vi "Common Path to Specific Path.vi"(10 "common path":string) -> (2 "specific path":path)   [LabVIEW 2020, in "NI_LVConfig.lvlib"]
uses:
  <vilib>/Utility/config.llb/NI_LVConfig.lvlib
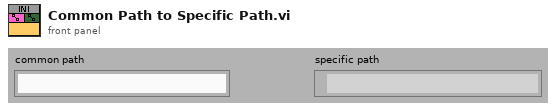
[diagram p1: front panel]
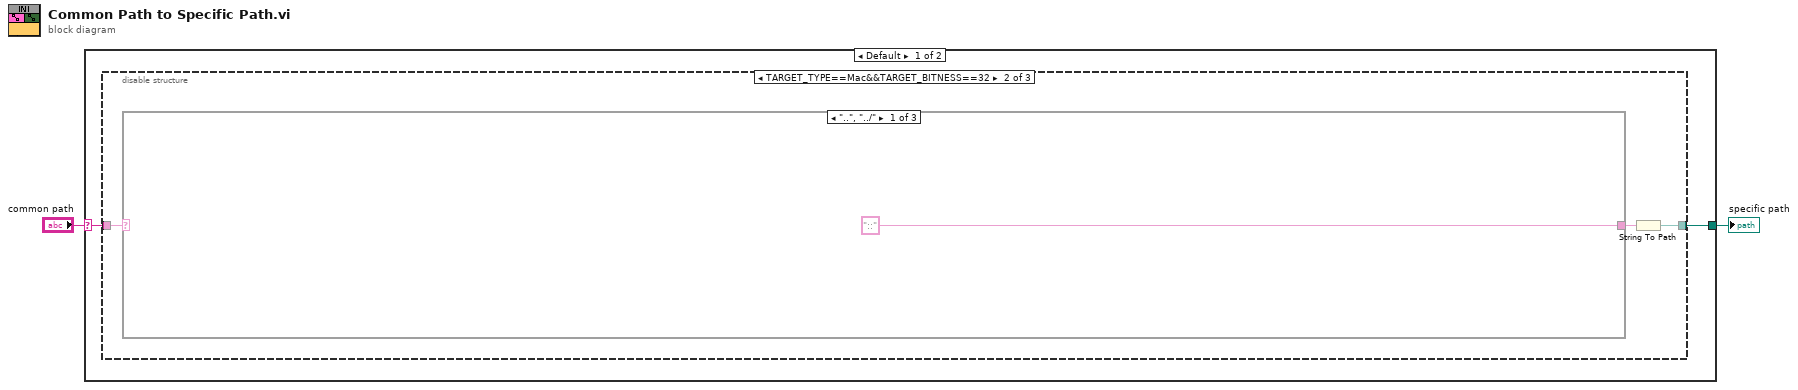
[diagram p0: block diagram]
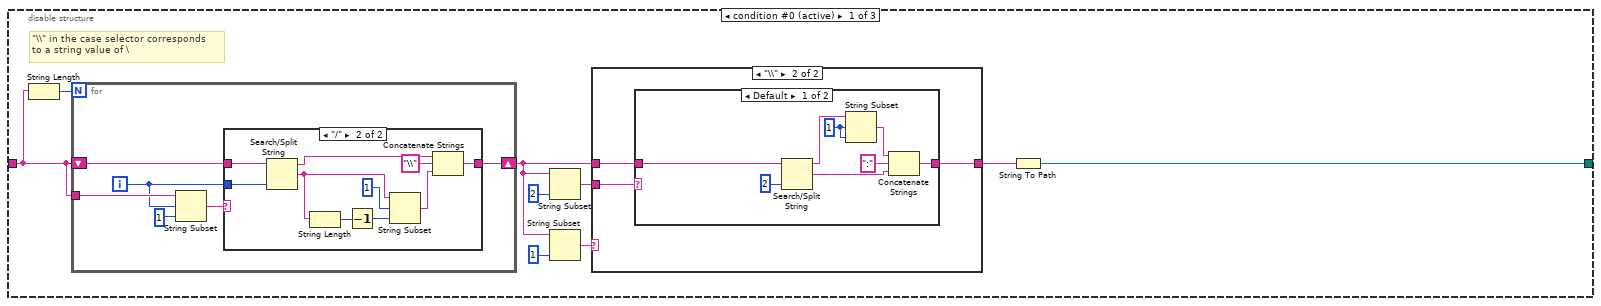
[diagram p2: hidden frame]
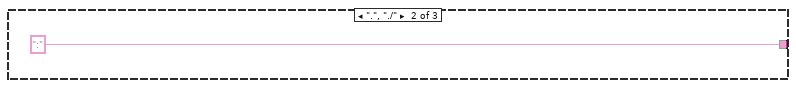
[diagram p6: hidden frame]
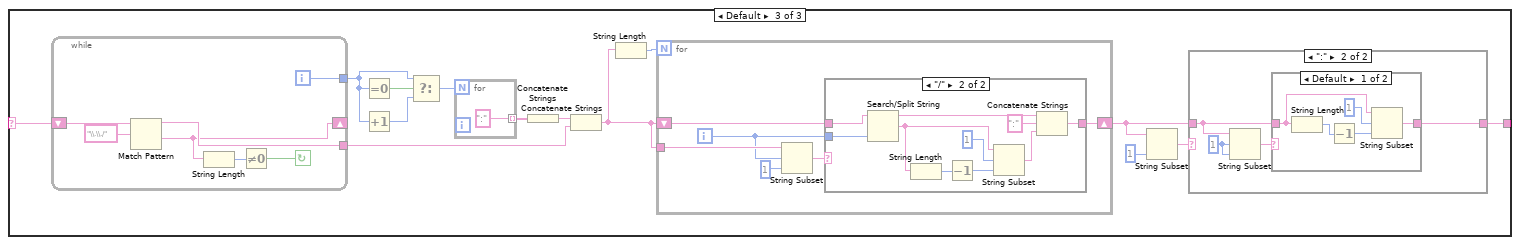
[diagram p7: hidden frame]
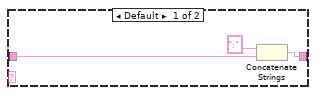
[diagram p9: hidden frame]
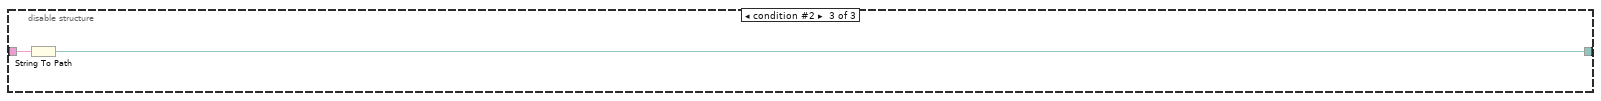
[diagram p11: hidden frame]
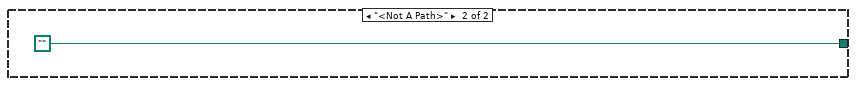
[diagram p12: hidden frame]
diagram:
  n1 = case shown="Default" "common path" {
    selector: "common path" -> [w4 _]
    tunnel: [w3 path "" ("Not A Path Constant")] -> w1
    frame Default {
      n2 = disable-structure "Conditional Disable Structure" shown="TARGET_TYPE==Mac&&TARGET_BITNESS==32" {
        disable-tunnel: w4 -> [w6 w45 w102]
        disable-tunnel: [w5 w44 w101] -> w3
        frame condition #0 (active) {
          # "\"\\\\\" in the case selector corresponds\nto a string value of \\"
          n3 = String Length(string=w6) -> (length=w10:i32)
          n4 = for {
            N: w10 -> [_]
            tunnel: w6 -> [w17]
            shift-right: [w18] -> w9
            shift-left: w6 -> [w19]
            i -> [w16]
            n5 = String Subset(string=w17, offset (0)=w16, length (rest)=1 ("length")) -> (substring=w14:string)
            n6 = case shown="\"/\"" w14 {
              tunnel: w19 -> [w20 w30]
              tunnel: w16 -> [_ w22]
              tunnel: [w20 w28] -> w18
              frame Default {
              }
              frame "/" {
                n7 = Search/Split String(string=w30, offset (0)=w22) -> (substring before match=w29:string, match + rest of string=w26:string)  [unwired: 2 out]
                n8 = String Length(string=w26) -> (length=w25:i32)
                n9 = Decrement(x=w25) -> (x-1=w24:i32)
                n10 = String Subset(string=w26, offset (0)=1, length (rest)=w24) -> (substring=w21:string)
                n11 = Concatenate Strings(w29, "\\" ("x"), w21) -> (w28:string)
              }
            }
          }
          n12 = String Subset(string=w9, length (rest)=2 ("length")) -> (substring=w7:string)  [unwired: 1 out]
          n13 = String Subset(string=w9, length (rest)=1 ("length")) -> (substring=w8:string)  [unwired: 1 out]
          n14 = case shown="\"\\\\\"" w8 {
            tunnel: w9 -> [w31 w34]
            tunnel: [w31 w33] -> w12
            tunnel: w7 -> [_ w32]
            frame Default {
            }
            frame "\\" {
              n15 = case shown="Default" w32 {
                tunnel: w34 -> [w42 w43]
                tunnel: [w36 w43] -> w33
                frame Default {
                  w35 = 1 ("offset (0)")
                  n16 = Search/Split String(string=w42, offset (0)=2) -> (substring before match=w40:string, match + rest of string=w37:string)  [unwired: 2 out]
                  n17 = String Subset(string=w40, offset (0)=w35, length (rest)=w35) -> (substring=w39:string)
                  n18 = Concatenate Strings(w39, ":", w37) -> (w36:string)
                }
                frame "\\\\" {
                  # "\"\\\\\\\\\" in the case selector corresponds\nto a string value of \\\\"
                }
              }
            }
          }
          n19 = String To Path(string=w12) -> (path=w5:path)
        }
        frame condition #1 {
          n20 = case shown="\"..\", \"../\"" w45 {
            selector: w45 -> [_ _ w52]
            tunnel: ["::" ":" w51] -> w46
            frame "..", "../" {
            }
            frame ".", "./" {
            }
            frame Default {
              n21 = while {
                tunnel: [w63] -> w60
                tunnel: [w65] -> w56
                shift-left: w52 -> [w68]
                shift-right: [w64] -> _
                i -> [w63]
                stop <- w66 continue-if-true
                n22 = Match Pattern(string=w68, regular expression="\\.\\./") -> (before substring=w65:string, after substring=w64:string)  [unwired: 3 out]
                n23 = String Length(string=w64) -> (length=w67:i32)
                n24 = Not Equal To 0?(x=w67) -> (x != 0?=w66:bool)
              }
              n25 = Equal To 0?(x=w60) -> (x = 0?=w61:bool)
              n26 = Increment(x=w60) -> (x+1=w59:i32)
              n27 = Select(t=w60, s=w61, f=w59) -> (s? t:f=w58:i32)
              n28 = for {
                N: w58 -> [_]
                tunnel: [":"] -> w57 mode=indexing
              }
              n29 = Concatenate Strings(w57) -> (w50:string)
              n30 = Concatenate Strings(w50, w56) -> (w54:string)
              n31 = String Length(string=w54) -> (length=w55:i32)
              n32 = for {
                N: w55 -> [_]
                tunnel: w54 -> [w73]
                shift-right: [w74] -> w49
                shift-left: w54 -> [w75]
                i -> [w72]
                n33 = String Subset(string=w73, offset (0)=w72, length (rest)=1 ("length")) -> (substring=w70:string)
                n34 = case shown="\"/\"" w70 {
                  tunnel: w75 -> [w76 w86]
                  tunnel: w72 -> [_ w79]
                  tunnel: [w76 w84] -> w74
                  frame Default {
                  }
                  frame "/" {
                    n35 = Search/Split String(string=w86, offset (0)=w79) -> (substring before match=w85:string, match + rest of string=w78:string)  [unwired: 2 out]
                    n36 = String Length(string=w78) -> (length=w82:i32)
                    n37 = Decrement(x=w82) -> (x-1=w81:i32)
                    n38 = String Subset(string=w78, offset (0)=1, length (rest)=w81) -> (substring=w77:string)
                    n39 = Concatenate Strings(w85, ":" ("x"), w77) -> (w84:string)
                  }
                }
              }
              n40 = String Subset(string=w49, length (rest)=1 ("length")) -> (substring=w53:string)  [unwired: 1 out]
              n41 = case shown="\":\"" w53 {
                tunnel: w49 -> [w90 w93]
                tunnel: [w89 w94] -> w51
                frame Default {
                  n42 = Concatenate Strings(":", w90) -> (w89:string)
                }
                frame ":" {
                  w92 = 1 ("length")
                  n43 = String Subset(string=w93, offset (0)=w92, length (rest)=w92) -> (substring=w91:string)
                  n44 = case shown="Default" w91 {
                    tunnel: w93 -> [w95 w100]
                    tunnel: [w96 w100] -> w94
                    frame Default {
                      n45 = String Length(string=w95) -> (length=w98:i32)
                      n46 = Decrement(x=w98) -> (x-1=w97:i32)
                      n47 = String Subset(string=w95, offset (0)=1, length (rest)=w97) -> (substring=w96:string)
                    }
                    frame ":" {
                    }
                  }
                }
              }
            }
          }
          n48 = String To Path(string=w46) -> (path=w44:path)
        }
        frame condition #2 {
          n49 = String To Path(string=w102) -> (path=w101:path)
        }
      }
    }
    frame "<Not A Path>" {
    }
  }
  "specific path" <- w1
